vi "Simulation Interface.vi"(8 "error in (no error)":errorcluster) -> (0 "error out":errorcluster)   [LabVIEW 2017]
doc: "Simulation Interface will be used to validate the Car Wash controller logic and algorithms."
uses:
  View Model/Controls/Interface.ctl
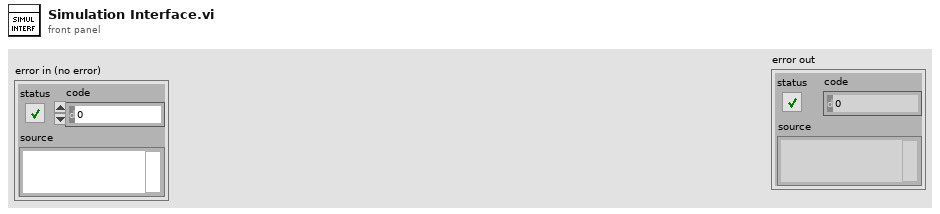
[diagram p1: front panel]
types:
  T1 = typedef "View Model.ctl" = cluster{"Shared Model":T2, "Error Model":T3, "DB Model":T4, "CNTRLR Model":T5}
  T2 = typedef "Shared Model.ctl" = cluster{"Stop":refnum<user-event>, "Stop DVR":refnum<data-value>}
  T3 = typedef "Error Model.ctl" = cluster{"Error Message":refnum<user-event>}
  T4 = typedef "Database Model.ctl" = cluster{"DB Message":refnum<user-event>, "DB Overhead DVR":refnum<data-value>}
  T5 = typedef "CNTRLR - Model.ctl" = cluster{"Message":refnum<user-event>, "Overhead DVR":refnum<data-value>, "Wash Entry":refnum<user-event>, "Out of Position":refnum<user-event>}
  T6 = typedef "Interface.ctl" = enum16{"Simulation", "Hardware"}
  T7 = enum32{"invalid app kind", "Development System", "Run Time System", "Student Edition", "Embedded LabVIEW", "Evaluation", "Custom"}
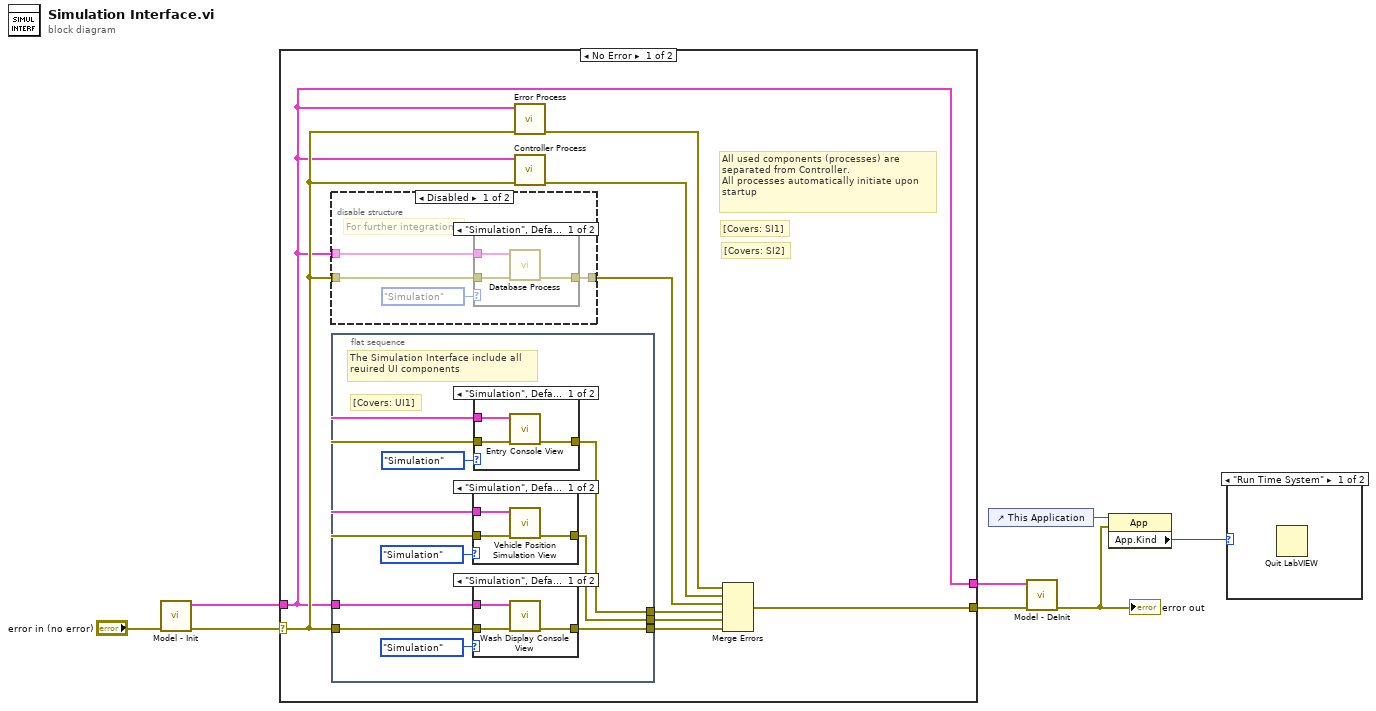
[diagram p0: block diagram]
diagram:
  n1 = call "Model - Init.vi"("error in (no error)"="error in (no error)") -> ("error out"=w7:errorcluster, "View Model"=w6:T1)  [unwired: 9 in]
  n2 = case shown="No Error" w7 {
    selector: w7 -> [w17 w48]
    tunnel: w6 -> [w9 w47]
    tunnel: [w10 w48] -> w5
    tunnel: [w9 w47] -> w4
    frame No Error {
      # "[Covers: SI2]"
      # "[Covers: SI1]"
      # "All used components (processes) are \nseparated from Controller.\nAll processes automatically initiate upon\nstartup"
      n3 = disable-structure shown="Disabled" {
        disable-tunnel: w9 -> [w40 _]
        disable-tunnel: w17 -> [w39 w46]
        disable-tunnel: [w38 w46] -> w13
        frame Disabled {
          # "For further integration"
          n4 = case shown="\"Simulation\", Default" Interface."Simulation" ("Interface") {
            tunnel: w40 -> [w44 _]
            tunnel: w39 -> [w43 w45]
            tunnel: [w42 w45] -> w38
            frame "Simulation", Default {
              n5 = call "Database Process.vi"("error in (no error)"=w43, "View Model"=w44) -> ("error out"=w42:errorcluster)  [unwired: 9 in]
            }
            frame "Hardware" {
            }
          }
        }
        frame Enabled {
        }
      }
      n6 = flat-sequence {
        tunnel: w17 -> [w22]
        tunnel: [w21] -> w16
        tunnel: [w20] -> w15
        tunnel: [w19] -> w14
        tunnel: w9 -> [w18]
        frame #0 {
          # "[Covers: UI1]"
          # "The Simulation Interface include all\nreuired UI components"
          n7 = case shown="\"Simulation\", Default" Interface."Simulation" ("Interface") {
            tunnel: w18 -> [w32 _]
            tunnel: w22 -> [w31 w33]
            tunnel: [w30 w33] -> w20
            frame "Simulation", Default {
              n8 = call "Vehicle Position Simulation View.vi"("error in (no error)"=w31, "View Model"=w32) -> ("error out"=w30:errorcluster)  [unwired: 9 in]
            }
            frame "Hardware" {
            }
          }
          n9 = case shown="\"Simulation\", Default" Interface."Simulation" ("Interface") {
            tunnel: w18 -> [w35 _]
            tunnel: w22 -> [w36 w37]
            tunnel: [w34 w37] -> w21
            frame "Simulation", Default {
              n10 = call "Wash Display Console View.vi"("error in (no error)"=w36, "View Model"=w35) -> ("error out"=w34:errorcluster)  [unwired: 9 in]
            }
            frame "Hardware" {
            }
          }
          n11 = case shown="\"Simulation\", Default" Interface."Simulation" ("Interface") {
            tunnel: w18 -> [w28 _]
            tunnel: w22 -> [w27 w29]
            tunnel: [w26 w29] -> w19
            frame "Simulation", Default {
              n12 = call "Entry Console View.vi"("error in (no error)"=w27, "View Model"=w28) -> ("error out"=w26:errorcluster)  [unwired: 9 in]
            }
            frame "Hardware" {
            }
          }
        }
      }
      n13 = call "Error Process.vi"("error in (no error)"=w17, "View Model"=w9) -> ("error out"=w11:errorcluster)  [unwired: 9 in]
      n14 = call "Controller Process.vi"("error in (no error)"=w17, "View Model"=w9) -> ("error out"=w12:errorcluster)  [unwired: 9 in]
      n15 = Merge Errors(w11, w12, w13, w14, w15, w16) -> (w10:errorcluster)
    }
    frame Error {
    }
  }
  n16 = control-ref of="This Application"() -> (w3:refnum<vi>)
  n17 = call "Model - DeInit.vi"("error in (no error)"=w5, "View Model"=w4) -> ("error out"=w1:errorcluster)  [unwired: 9 in]
  "error out" <- w1
  n18 = property class="App"(reference=w3, error in=w1) -> ("App.Kind"=w2:T7)  [unwired: 2 out]
  n19 = case shown="\"Run Time System\"" w2 {
    frame "Run Time System" {
      n20 = Quit LabVIEW() -> ()  [unwired: 1 in]
    }
    frame "Development System", Default {
    }
  }
